vi "async output data method.vi"(6 "transfer specification in":T1[](array[typedef]), 7 "engine tag data in":T3, 8 "error in":errorcluster, 11 "async exec in":T4) -> (0 "error out":errorcluster, 3 "async exec out":T4, 4 "transfer specification out":T1[](array[typedef]), 5 "engine tag data out":T3)   [LabVIEW 2013, in "main engine.lvlib"]
uses:
  main engine/main engine.lvlib
  asynchronous executor reference.ctl
  async message to executor.ctl
  Runtime/async command notification.ctl
  <vilib>/NI/Tag Bus/table/data table.ctl
  Runtime/async error info.ctl
  <vilib>/NI/Tag Bus Module Framework/runtime/error classification.ctl
  <vilib>/NI/Tag Bus/table/transfer specification.ctl
  <vilib>/NI/Tag Bus/tag/Data Type.ctl
  <vilib>/NI/Tag Bus/table/data table.lvlib
  <vilib>/NI/Tag Bus/tag/tag descriptor.lvclass
  <vilib>/NI/Tag Bus Module Framework/runtime/TBM module execution interface.lvclass
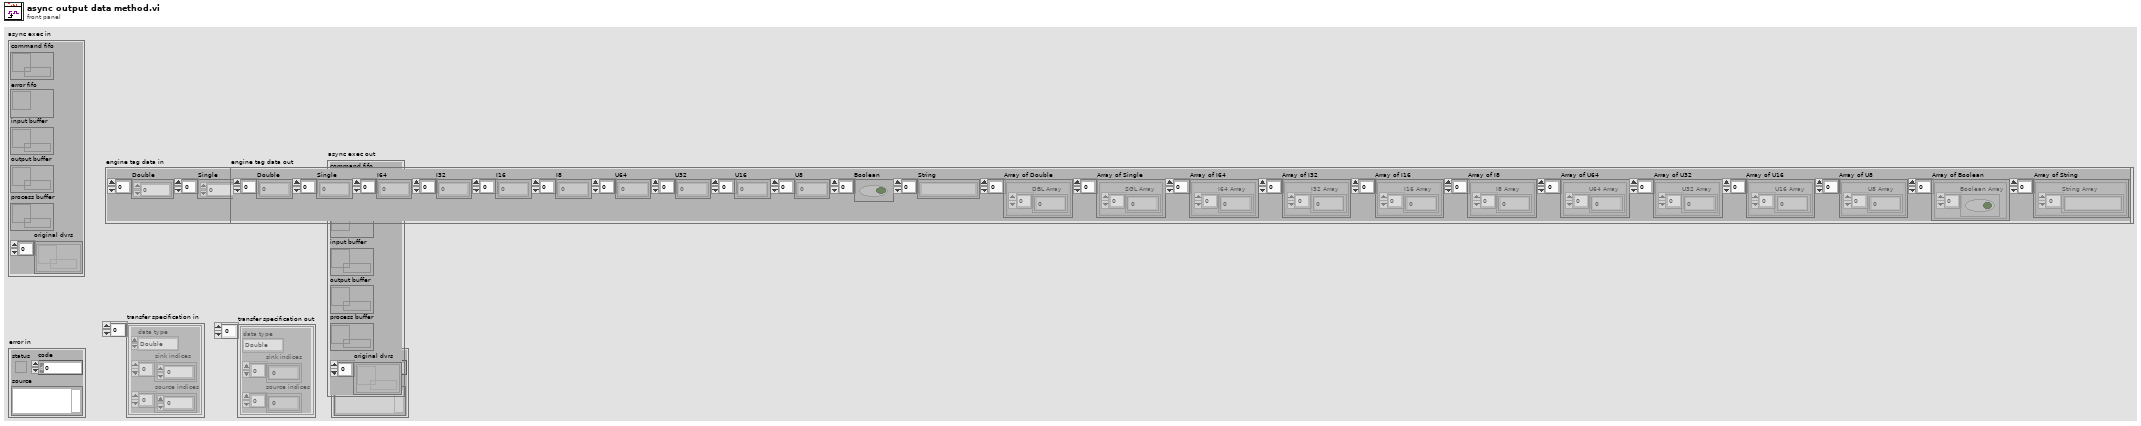
[diagram p1: front panel]
types:
  T1 = typedef "tag bus.lvlib/data table.lvlib/transfer specification.ctl" = cluster{"data type":T2, "sink indices":i32[], "source indices":i32[]}
  T2 = typedef "tag bus.lvlib/tag descriptor.lvclass/Data Type.ctl" = enum16{"Double", "Single", "I64", "I32", "I16", "I8", "U64", "U32", "U16", "U8", "Boolean", "String", "Array of Double", "Array of Single", "Array of I64", "Array of I32", "Array of I16", "Array of I8", "Array of U64", "Array of U32", "Array of U16", "Array of U8", "Array of Boolean", "Array of String"}
  T3 = typedef "tag bus.lvlib/data table.lvlib/data table.ctl" = cluster{"Double":dbl[], "Single":sgl[], "I64":i64[], "I32":i32[], "I16":i16[], "I8":i8[], "U64":u64[], "U32":u32[], "U16":u16[], "U8":u8[], "Boolean":bool[], "String":string[], "Array of Double":cluster{"DBL Array":dbl[]}[], "Array of Single":cluster{"SGL Array":sgl[]}[], "Array of I64":cluster{"I64 Array":i64[]}[], "Array of I32":cluster{"I32 Array":i32[]}[], "Array of I16":cluster{"I16 Array":i16[]}[], "Array of I8":cluster{"I8 Array":i8[]}[], "Array of U64":cluster{"U64 Array":u64[]}[], "Array of U32":cluster{"U32 Array":u32[]}[], "Array of U16":cluster{"U16 Array":u16[]}[], "Array of U8":cluster{"U8 Array":u8[]}[], "Array of Boolean":cluster{"Boolean Array":bool[]}[], "Array of String":cluster{"String Array":string[]}[]}
  T4 = typedef "main engine.lvlib/asynchronous executor reference.ctl" = cluster{"command fifo":refnum<k33>, "error fifo":refnum<k33>, "input buffer":refnum<k33>, "output buffer":refnum<k33>, "process buffer":refnum<k33>, "original dvrs":refnum<data-value>[]}
  T5 = typedef "main engine.lvlib/async command notification.ctl" = enum16{"stop", "input", "process", "output"}
  T6 = typedef "main engine.lvlib/async message to executor.ctl" = cluster{"command":T5, "data 1 (i,o,pp)":refnum<data-value>, "data 2 (pr)":refnum<data-value>, "user value":u64}
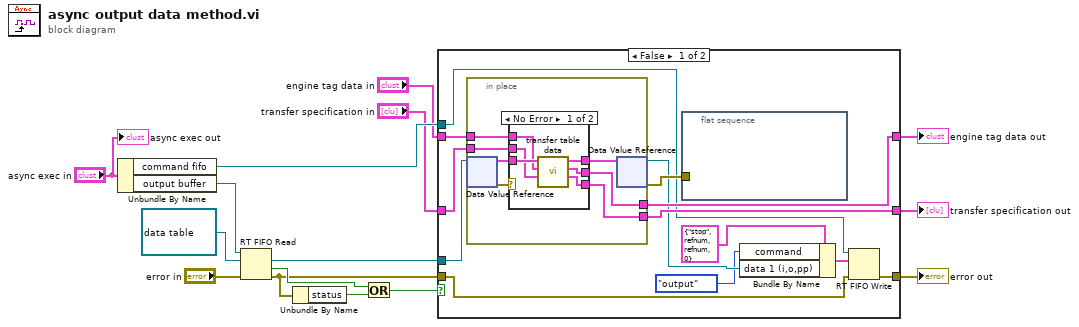
[diagram p0: block diagram]
diagram:
  n1 = Unbundle By Name("async exec in") -> ("command fifo"=w9:refnum<k33>, "output buffer"=w15:refnum<k33>)
  n2 = RT FIFO Read(0:w15, 1:refnum<data-value> refnum ("element"), 3:"error in") -> (9:w14:refnum<data-value>, 10:w13:bool, 11:w10:errorcluster)  [unwired: 1 in, 2 out]
  n3 = Unbundle By Name(w10) -> ("status"=w12:bool)
  n4 = Or(x=w13, y=w12) -> (x .or. y?=w8:bool)
  n5 = case shown="False" w8 {
    tunnel: "engine tag data in" -> [w28 w46]
    tunnel: [w27 w46] -> w4
    tunnel: w14 -> [w25 _]
    tunnel: [w24 w47] -> w1
    tunnel: "transfer specification in" -> [w23 w47]
    tunnel: [w21 w45] -> w5
    tunnel: w10 -> [w22 w45]
    tunnel: w9 -> [w20 _]
    frame False {
      n6 = in-place {
        in-place-border: w28 -> [w35]
        in-place-border: [w34] -> w27
        in-place-border: [w32] -> w24
        in-place-border: w23 -> [w31]
        n7 = in-place-dvr #1(w25) -> (w30:T3, w33:errorcluster)
        n8 = case shown="No Error" w33 {
          tunnel: w35 -> [w38 w43]
          tunnel: [w39 w43] -> w34
          tunnel: [w36 w44] -> w32
          tunnel: w31 -> [w37 w44]
          tunnel: w30 -> [w41 w42]
          tunnel: [w40 w42] -> w29
          frame No Error {
            n9 = call <vilib>:"transfer table data.vi"("transfer specification in"=w37, "data table source in"=w38, "data table sink in"=w41) -> ("transfer specification out"=w36:T1[], "data table source out"=w39:T3, "data table sink out"=w40:T3)  [unwired: 6 in]
          }
          frame Error {
          }
        }
        n10 = in-place-dvr #1(w29) -> (w17:refnum<data-value>, w26:errorcluster)
      }
      n11 = flat-sequence {
        tunnel: w26 -> [_]
        frame #0 {
        }
      }
      n12 = Bundle By Name(cluster=T6 {"command"=enum."stop", "data 1 (i,o,pp)"=refnum, "data 2 (pr)"=refnum, "user value"=0} ("element"), "command"=async_command_notification."output", "data 1 (i,o,pp)"=w17) -> (w18:T6)
      n13 = RT FIFO Write(0:w20, 1:w18, 3:w22) -> (11:w21:errorcluster)  [unwired: 2 in, 3 out]
    }
    frame True {
    }
  }
  "error out" <- w5
  "engine tag data out" <- w4
  "transfer specification out" <- w1
  "async exec out" <- "async exec in"
